vi "PRL Remote.vi"(8 "error in (no error)":errorcluster, 11 "Action":T1(ring)) -> (0 "error out":errorcluster, 1 "Connected":bool, 2 "Configuration File Received":bool, 3 "Buffer Active":bool, 4 "Number of bad dt":u64, 5 "Queue Active":bool)   [LabVIEW 2013, in "PMU Recorder Light.lvlib"]
doc: "Sends commands to the PRL"
uses:
  PMU Recorder Light.lvlib
  <vilib>/Utility/error.llb/DialogType.ctl
panel:
  # "INPUT"
  # "INTERMEDIATE"
  # "OUTPUT"
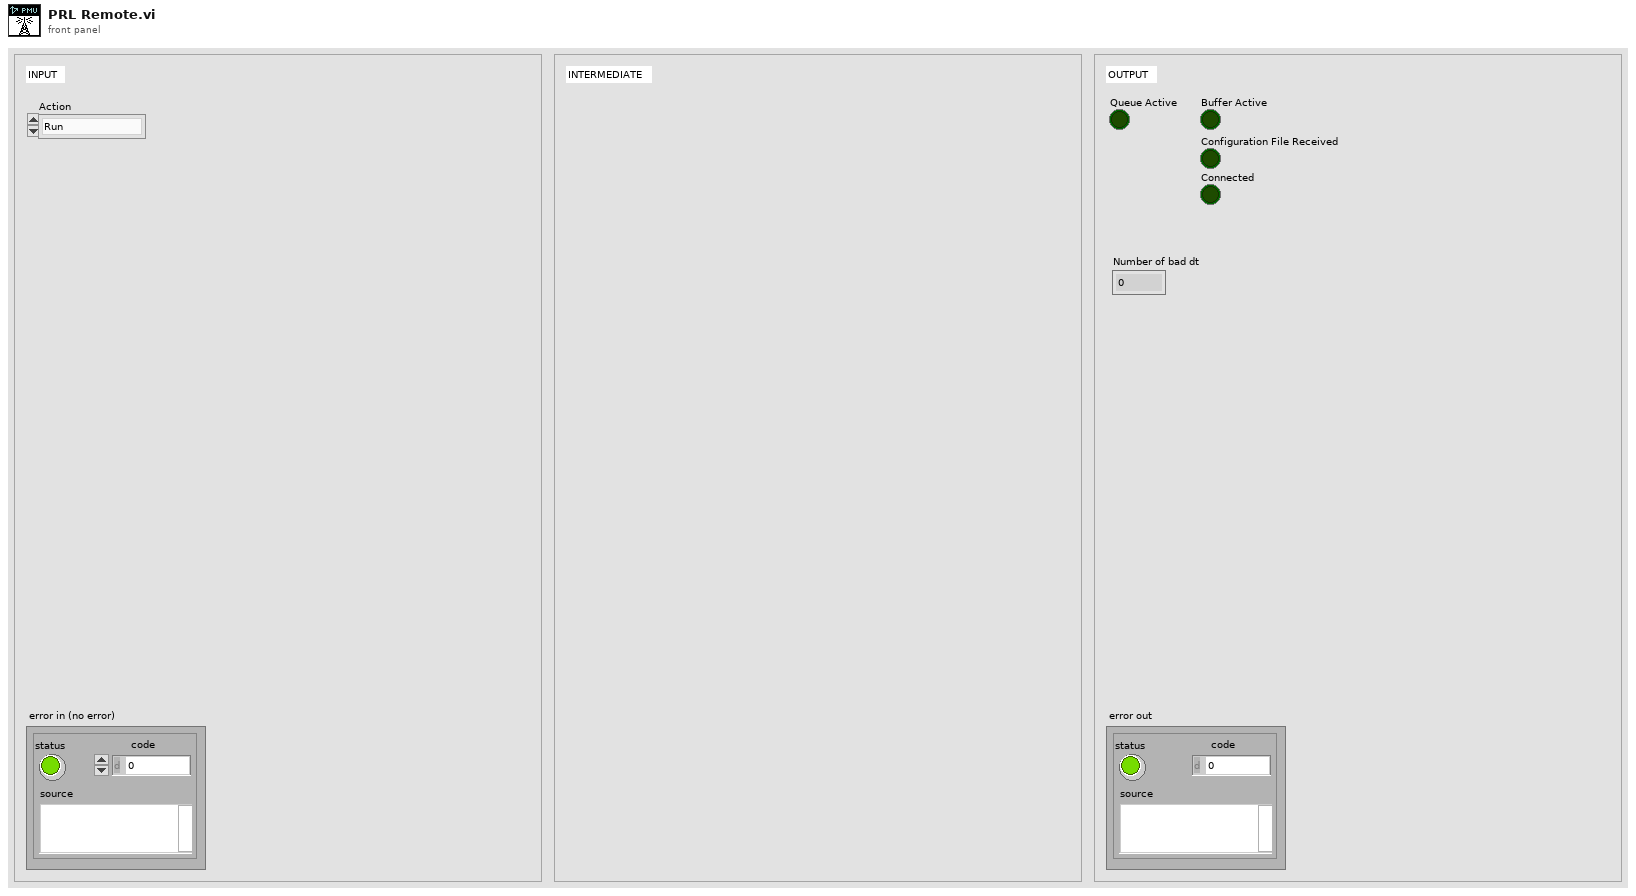
[diagram p1: front panel]
types:
  T1 = enum16{"Run", "Startup", "Get Status", "Pause", "Continue", "Shutdown", "Abort", "Open Panel", "Close Panel"}
  T2 = enum32{"Invalid", "Standard", "Closed", "Hidden", "Minimized", "Maximized"}
  T3 = typedef "DialogType.ctl" = u16
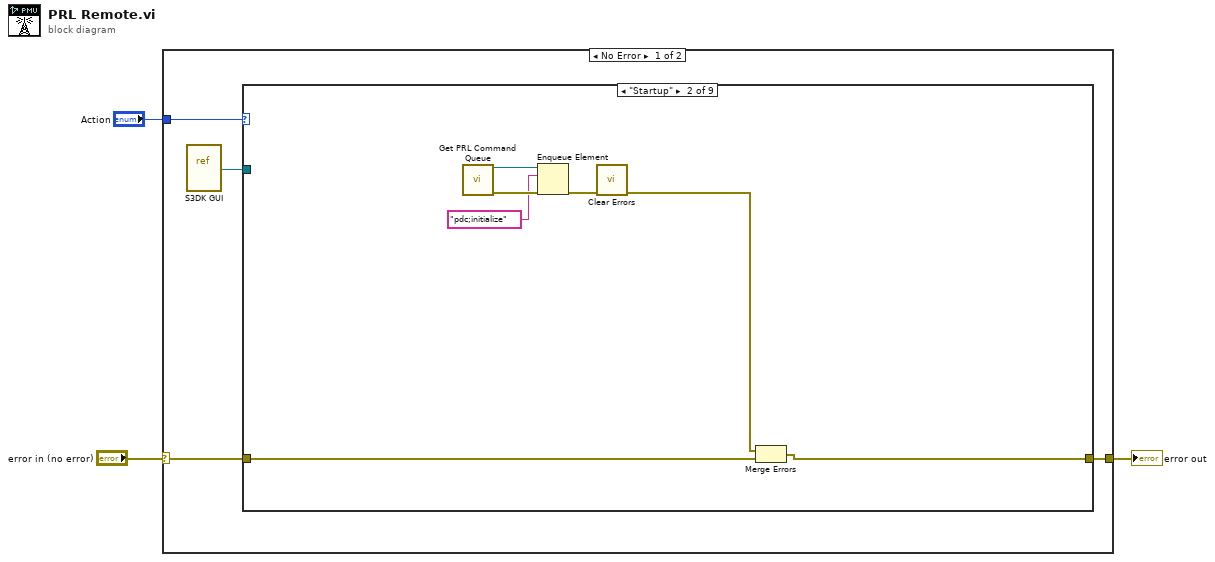
[diagram p0: block diagram]
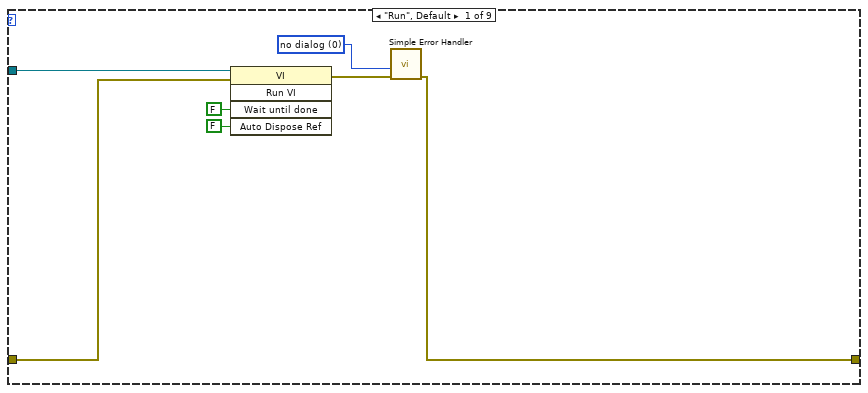
[diagram p2: hidden frame]
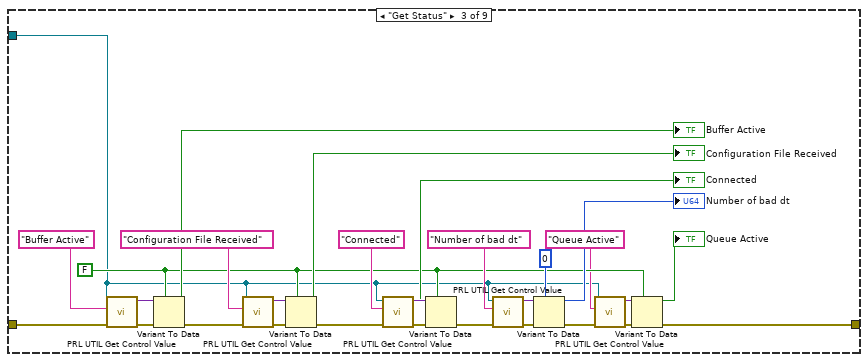
[diagram p3: hidden frame]
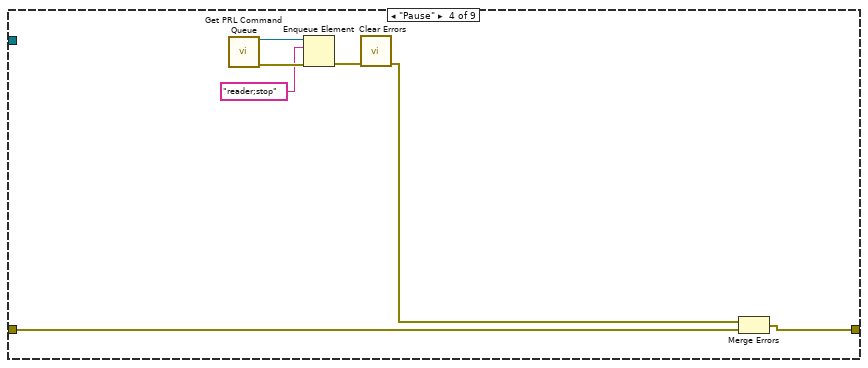
[diagram p4: hidden frame]
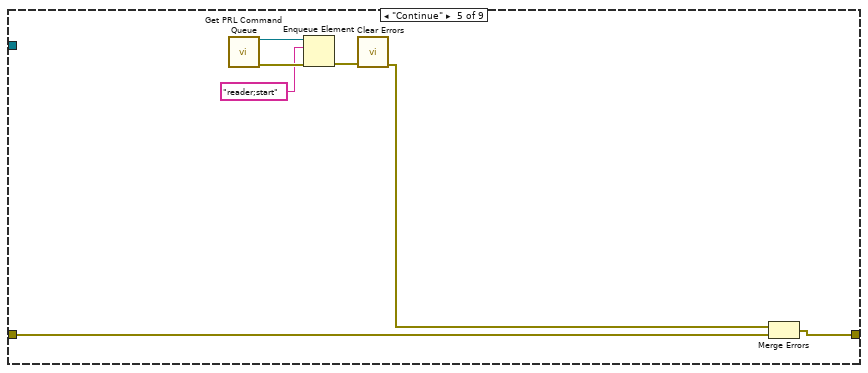
[diagram p5: hidden frame]
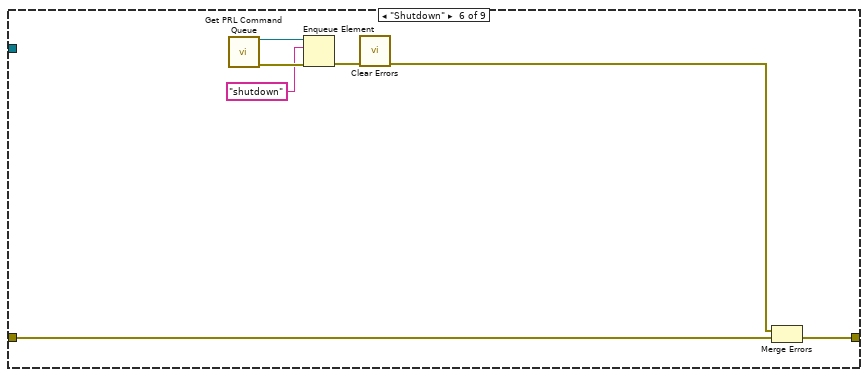
[diagram p6: hidden frame]
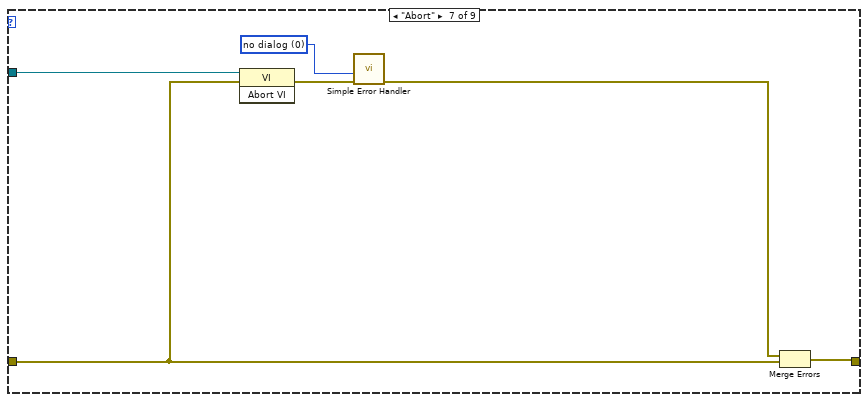
[diagram p7: hidden frame]
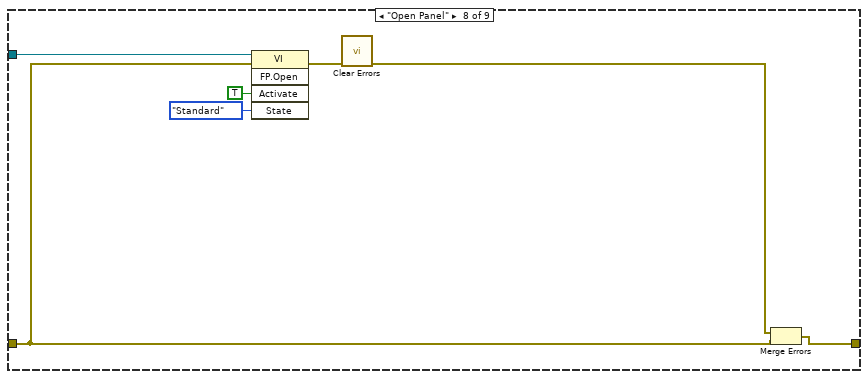
[diagram p8: hidden frame]
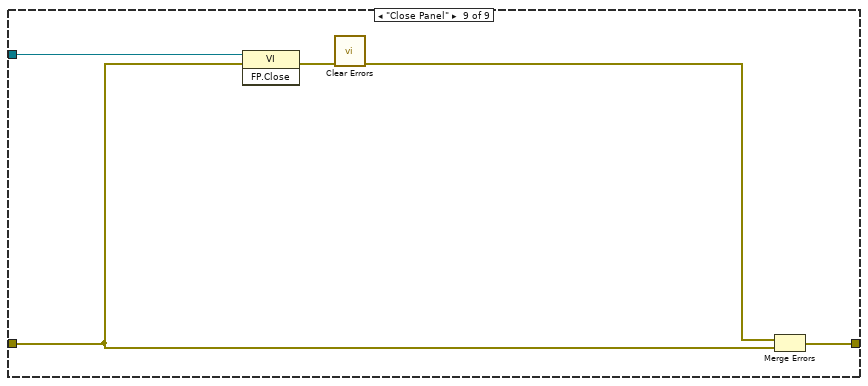
[diagram p9: hidden frame]
diagram:
  n1 = case shown="No Error" "error in (no error)" {
    selector: "error in (no error)" -> [w5 w90]
    tunnel: "Action" -> [w6 _]
    tunnel: [w4 w90] -> w1
    frame No Error {
      n2 = vi-ref "S3DK GUI.vi"() -> (w7:refnum<vi>)
      n3 = case shown="\"Startup\"" w6 {
        tunnel: w7 -> [w14 _ w22 _ _ _ w77 w84 w89]
        tunnel: w5 -> [w9 w17 w25 w52 w59 w67 w72 w79 w86]
        tunnel: [w8 w16 w23 w51 w58 w65 w73 w80 w87] -> w4
        frame "Run", Default {
          w10 = T3 0 items=["no dialog", "OK message", "continue or stop message", "OK message + warnings", "continue/stop + warnings"] ("type of dialog (OK msg:1)")
          n4 = invoke class="VI" method="Run VI"(reference=w14, error in=w9, "Wait until done"=FALSE ("Wait Until Done"), "Auto Dispose Ref"=FALSE ("Auto Dispose Reference")) -> (error out=w11:errorcluster)  [unwired: 1 in, 4 out]
          n5 = call <vilib>:"Simple Error Handler.vi"("type of dialog (OK msg:1)"=w10, "error in (no error)"=w11) -> ("error out"=w8:errorcluster)  [unwired: 3 in, 4 out]
        }
        frame "Startup" {
          n6 = call "Get PRL Command Queue.vi"() -> ("error out"=w20:errorcluster, "PRL Command Queue"=w21:refnum<queue>)  [unwired: 10 in]
          n7 = Enqueue Element(queue=w21, element="pdc;initialize", error in (no error)=w20) -> (error out=w18:errorcluster)  [unwired: 1 in, 2 out]
          n8 = call <vilib>:"Clear Errors.vi"("error in (no error)"=w18) -> ("error out"=w15:errorcluster)  [unwired: 5 in, 1 out]
          n9 = Merge Errors(w15, w17) -> (w16:errorcluster)
        }
        frame "Get Status" {
          w29 = FALSE
          n10 = call "PRL UTIL Get Control Value.vi"("error in (no error)"=w25, "Control Name"="Buffer Active", "VI Reference"=w22) -> ("error out"=w46:errorcluster, "Value"=w47:variant)  [unwired: 7 in]
          n11 = Variant To Data(error in=w46, type=w29, Variant=w47) -> (data=→"Buffer Active":bool, error out=w45:errorcluster)
          n12 = call "PRL UTIL Get Control Value.vi"("error in (no error)"=w45, "Control Name"="Configuration File Received", "VI Reference"=w22) -> ("error out"=w44:errorcluster, "Value"=w43:variant)  [unwired: 7 in]
          n13 = Variant To Data(error in=w44, type=w29, Variant=w43) -> (data=→"Configuration File Received":bool, error out=w37:errorcluster)
          n14 = call "PRL UTIL Get Control Value.vi"("error in (no error)"=w37, "Control Name"="Connected", "VI Reference"=w22) -> ("error out"=w41:errorcluster, "Value"=w42:variant)  [unwired: 7 in]
          n15 = Variant To Data(error in=w41, type=w29, Variant=w42) -> (data=→"Connected":bool, error out=w35:errorcluster)
          n16 = call "PRL UTIL Get Control Value.vi"("error in (no error)"=w35, "Control Name"="Number of bad dt", "VI Reference"=w22) -> ("error out"=w33:errorcluster, "Value"=w34:variant)  [unwired: 7 in]
          n17 = Variant To Data(error in=w33, type=u64 0 ("Number of bad dt"), Variant=w34) -> (data=→"Number of bad dt":u64, error out=w30:errorcluster)
          n18 = call "PRL UTIL Get Control Value.vi"("error in (no error)"=w30, "Control Name"="Queue Active", "VI Reference"=w22) -> ("error out"=w24:errorcluster, "Value"=w28:variant)  [unwired: 7 in]
          n19 = Variant To Data(error in=w24, type=w29, Variant=w28) -> (data=→"Queue Active":bool, error out=w23:errorcluster)
        }
        frame "Pause" {
          n20 = call "Get PRL Command Queue.vi"() -> ("error out"=w56:errorcluster, "PRL Command Queue"=w57:refnum<queue>)  [unwired: 10 in]
          n21 = Enqueue Element(queue=w57, element="reader;stop", error in (no error)=w56) -> (error out=w54:errorcluster)  [unwired: 1 in, 2 out]
          n22 = call <vilib>:"Clear Errors.vi"("error in (no error)"=w54) -> ("error out"=w53:errorcluster)  [unwired: 5 in, 1 out]
          n23 = Merge Errors(w53, w52) -> (w51:errorcluster)
        }
        frame "Continue" {
          n24 = call "Get PRL Command Queue.vi"() -> ("error out"=w63:errorcluster, "PRL Command Queue"=w64:refnum<queue>)  [unwired: 10 in]
          n25 = Enqueue Element(queue=w64, element="reader;start", error in (no error)=w63) -> (error out=w61:errorcluster)  [unwired: 1 in, 2 out]
          n26 = call <vilib>:"Clear Errors.vi"("error in (no error)"=w61) -> ("error out"=w60:errorcluster)  [unwired: 5 in, 1 out]
          n27 = Merge Errors(w60, w59) -> (w58:errorcluster)
        }
        frame "Shutdown" {
          n28 = call "Get PRL Command Queue.vi"() -> ("error out"=w70:errorcluster, "PRL Command Queue"=w71:refnum<queue>)  [unwired: 10 in]
          n29 = Enqueue Element(queue=w71, element="shutdown", error in (no error)=w70) -> (error out=w68:errorcluster)  [unwired: 1 in, 2 out]
          n30 = call <vilib>:"Clear Errors.vi"("error in (no error)"=w68) -> ("error out"=w66:errorcluster)  [unwired: 5 in, 1 out]
          n31 = Merge Errors(w66, w67) -> (w65:errorcluster)
        }
        frame "Abort" {
          w75 = T3 0 items=["no dialog", "OK message", "continue or stop message", "OK message + warnings", "continue/stop + warnings"] ("type of dialog (OK msg:1)")
          n32 = invoke class="VI" method="Abort VI"(reference=w77, error in=w72) -> (error out=w76:errorcluster)  [unwired: 1 in, 2 out]
          n33 = call <vilib>:"Simple Error Handler.vi"("type of dialog (OK msg:1)"=w75, "error in (no error)"=w76) -> ("error out"=w74:errorcluster)  [unwired: 3 in, 4 out]
          n34 = Merge Errors(w74, w72) -> (w73:errorcluster)
        }
        frame "Open Panel" {
          n35 = invoke class="VI" method="FP.Open"(reference=w84, error in=w79, "Activate"=TRUE ("Activate?"), "State"=T2."Standard") -> (error out=w81:errorcluster)  [unwired: 1 in, 4 out]
          n36 = call <vilib>:"Clear Errors.vi"("error in (no error)"=w81) -> ("error out"=w78:errorcluster)  [unwired: 5 in, 1 out]
          n37 = Merge Errors(w78, w79) -> (w80:errorcluster)
        }
        frame "Close Panel" {
          n38 = invoke class="VI" method="FP.Close"(reference=w89, error in=w86) -> (error out=w88:errorcluster)  [unwired: 1 in, 2 out]
          n39 = call <vilib>:"Clear Errors.vi"("error in (no error)"=w88) -> ("error out"=w85:errorcluster)  [unwired: 5 in, 1 out]
          n40 = Merge Errors(w85, w86) -> (w87:errorcluster)
        }
      }
    }
    frame Error {
    }
  }
  "error out" <- w1
